vi "crop.vi"(0 "Image in":T1, 1 "left":i32, 2 "right":i32, 3 "top":i32, 4 "bottom":i32, 5 "error in (no error)":errorcluster) -> (14 "Image out":T1, 19 "error out":errorcluster)   [LabVIEW 2023, in "Vision.lvlib"]
uses:
  Vision.lvlib
  <vilib>/vision/Image Controls.llb/IMAQ Image.ctl
  bin/Vision.dll
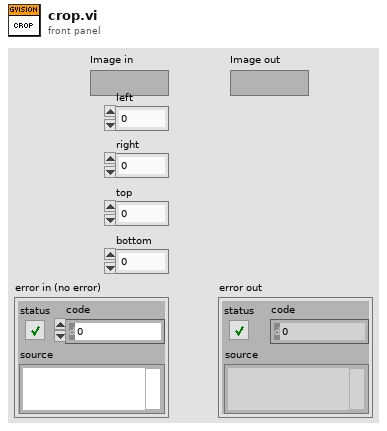
[diagram p1: front panel]
types:
  T1 = typedef "IMAQ Image.ctl" = refnum<image>
  T2 = enum32{"Map Pixel Pointer", "Unmap Pixel Pointer", "Get Pixels Infos"}
  T3 = typedef "Image Type" = u32
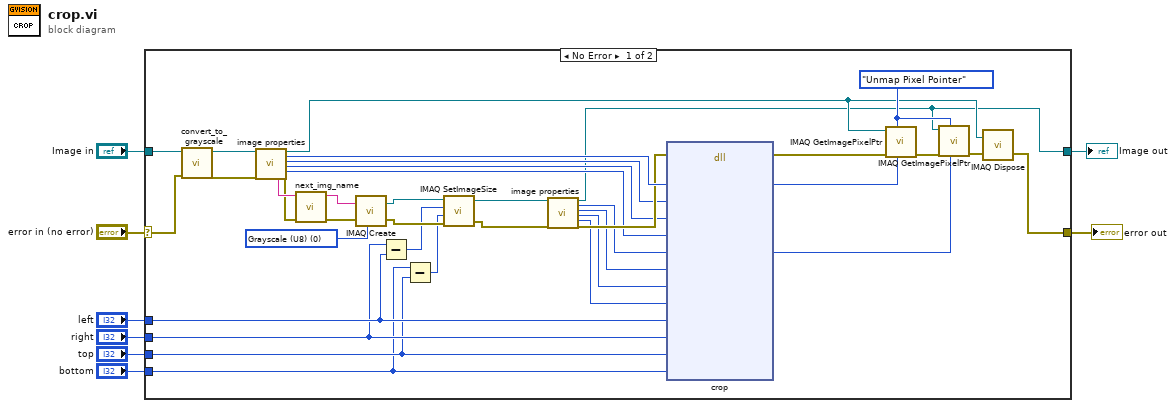
[diagram p0: block diagram]
diagram:
  n1 = case shown="No Error" "error in (no error)" {
    selector: "error in (no error)" -> [w38 w47]
    tunnel: "Image in" -> [w39 w46]
    tunnel: [w45 w47] -> w6
    tunnel: [w13 w46] -> w5
    tunnel: "left" -> [w20 _]
    tunnel: "right" -> [w19 _]
    tunnel: "top" -> [w18 _]
    tunnel: "bottom" -> [w17 _]
    frame No Error {
      w40 = T2."Unmap Pixel Pointer" ("Function")
      w44 = T3 0 items=["Grayscale (U8)", "Grayscale (I16)", "Grayscale (SGL)", "Complex (CSG)", "RGB (U32)", "HSL (U32)", "RGB (U64)", "Grayscale (U16)"] ("Image Type")
      n2 = call "convert_to_grayscale.vi"("error in (no error)"=w38, "Image in"=w39) -> ("error out"=w36:errorcluster, "Image out"=w37:T1)  [unwired: 8 in]
      n3 = call "image properties.vi"("Image in"=w37, "error in (no error)"=w36) -> ("Image Name"=w12:string, "Image out"=w14:T1, "Pixel Pointer out"=w29:u64, "Line Width"=w27:i32, "X Resolution"=w26:i32, "Y Resolution"=w25:i32, "error out"=w10:errorcluster)  [unwired: 10 in, 1 out]
      n4 = call "next_img_name.vi"("error in (no error)"=w10, "name in"=w12) -> ("error out"=w9:errorcluster, "name out"=w11:string)  [unwired: 8 in]
      n5 = call "IMAQ Create"("Image Name"=w11, "Image Type"=w44, "error in (no error)"=w9) -> ("New Image"=w35:T1, "error out"=w34:errorcluster)  [unwired: 2 in]
      n6 = Subtract(x=w19, y=w20) -> (x-y=w33:i32)
      n7 = Subtract(x=w17, y=w18) -> (x-y=w32:i32)
      n8 = call "IMAQ SetImageSize"("error in (no error)"=w34, "Y Resolution"=w32, "X Resolution"=w33, "Image"=w35) -> ("error out"=w30:errorcluster, "Image Out"=w31:T1)  [unwired: 1 in]
      n9 = call "image properties.vi"("Image in"=w31, "error in (no error)"=w30) -> ("Image out"=w13:T1, "Pixel Pointer out"=w24:u64, "Line Width"=w23:i32, "X Resolution"=w22:i32, "Y Resolution"=w21:i32, "error out"=w28:errorcluster)  [unwired: 10 in, 2 out]
      n10 = dll-call lib="C:/Users/cfangmeier3/Desktop/nebraska-silicon-lab/pixel-gantry-control/Gantry/Shared Components/bin/Vision.dll" fn="crop"(error in=w28, "src_imgPtr"=w29, "src_imgLineWidth"=w27, "src_imgWidth"=w26, "src_imgHeight"=w25, "dst_imgPtr"=w24, "dst_imgLineWidth"=w23, "dst_imgWidth"=w22, "dst_imgHeight"=w21, "left"=w20, "right"=w19, "top"=w18, "bottom"=w17) -> (error out=w42:errorcluster, "src_imgPtr"=w16:u64, "dst_imgPtr"=w15:u64)  [unwired: 13 in, 1 out]
      n11 = call "IMAQ GetImagePixelPtr"("Pixel Pointer in"=w16, "Function"=w40, "error in (no error)"=w42, "Image"=w14) -> ("error out"=w43:errorcluster)  [unwired: 2 in, 5 out]
      n12 = call "IMAQ GetImagePixelPtr"("Pixel Pointer in"=w15, "Function"=w40, "error in (no error)"=w43, "Image"=w13) -> ("error out"=w41:errorcluster)  [unwired: 2 in, 5 out]
      n13 = call "IMAQ Dispose"("Image"=w14, "error in (no error)"=w41) -> ("error out"=w45:errorcluster)  [unwired: 4 in]
    }
    frame Error {
    }
  }
  "Image out" <- w5
  "error out" <- w6
